vi "Modbus Slave Simple.vi"() -> ()   [LabVIEW 2017]
uses:
  <vilib>/NI/Modbus Library/API/Wrapper/Create Serial Slave.vi
  <vilib>/NI/Modbus Library/API/Slave/Modbus Slave.lvclass
  <vilib>/NI/Modbus Library/API/Wrapper/API Main.lvlib
panel:
  out "Array 5":errorcluster[](array[cluster])
  in  "Inputs":T1(array[cluster])=[{"Inputs"=[0, 0, 0, 0], "Address"=0, "Number"=4}] {"Inputs" scale=0.0..65535.0}
  out "error out":errorcluster
  in  "Stop Button":bool
  in  "Start":bool
  out "Array 4":errorcluster[](array[cluster])
  out "Array 3":errorcluster[](array[cluster])
  out "Array 2":errorcluster[](array[cluster])
  out "Array":errorcluster[](array[cluster])
  in  "Write Holding Reg":T2(array[cluster])=[{"Registers"=[], "Address"=0, "Number"=2}]
  in  "Read Holding Reg":T2(array[cluster])=[{"Registers"=[0, 0], "Address"=0, "Number"=2}]
  in  "Discrete Inputs":T3(array[cluster])=[{"Inputs"=[TRUE, FALSE, TRUE, FALSE], "Address"=0, "Number"=4}]
  in  "Coils":T4(array[cluster])=[{"Coils"=[TRUE, TRUE, TRUE, TRUE, TRUE, FALSE, FALSE, FALSE], "Address"=0, "Number"=8}] {"Address" format="%x"}
  in  "Update Period(ms)":u64=200
  in  "baud rate":u32=9600
  in  "VISA resource name":refnum<visa-resource-name>="COM14"
  in  "unit ID":u8=1
  in  "serial type":enum16{"RTU", "ASCII"}(ring)=enum."ASCII"
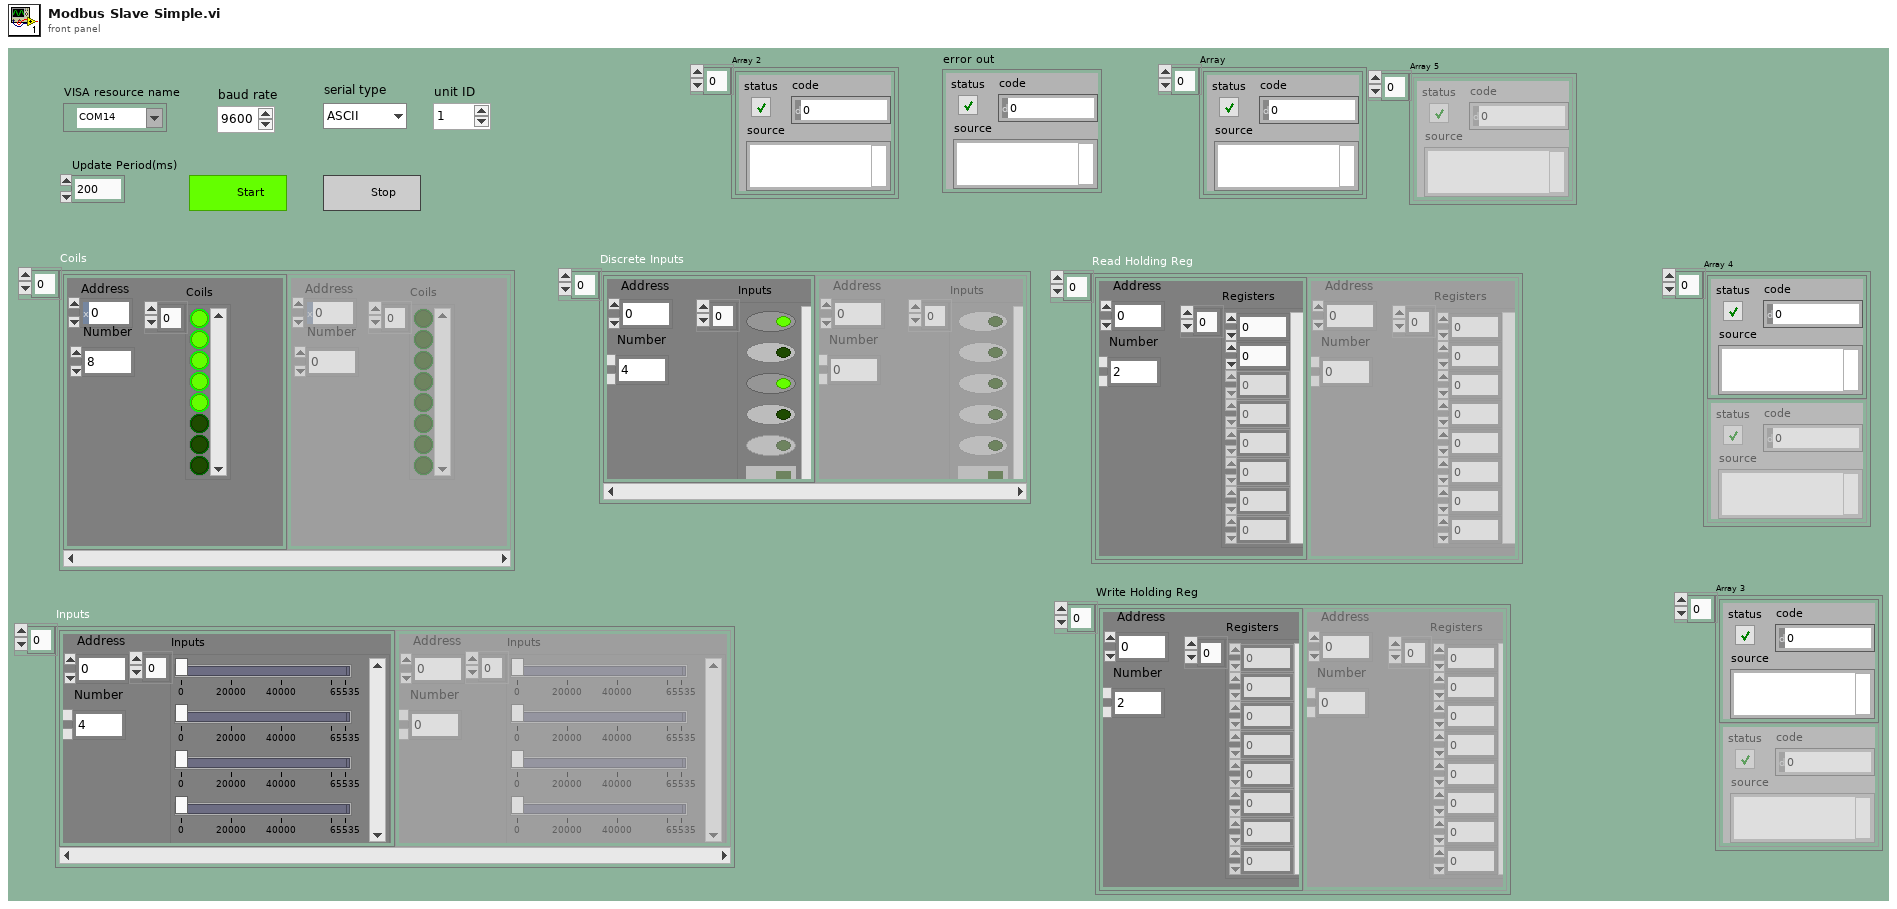
[diagram p1: front panel]
types:
  T1 = cluster{"Inputs":u16[], "Address":u16, "Number":u16}[]
  T2 = cluster{"Registers":u16[], "Address":u16, "Number":u16}[]
  T3 = cluster{"Inputs":bool[], "Address":u16, "Number":u16}[]
  T4 = cluster{"Coils":bool[], "Address":u16, "Number":u16}[]
  T5 = cluster{"Coils":bool[], "Address":u16, "Number":u16}
  T6 = cluster{"Registers":u16[], "Address":u16, "Number":u16}
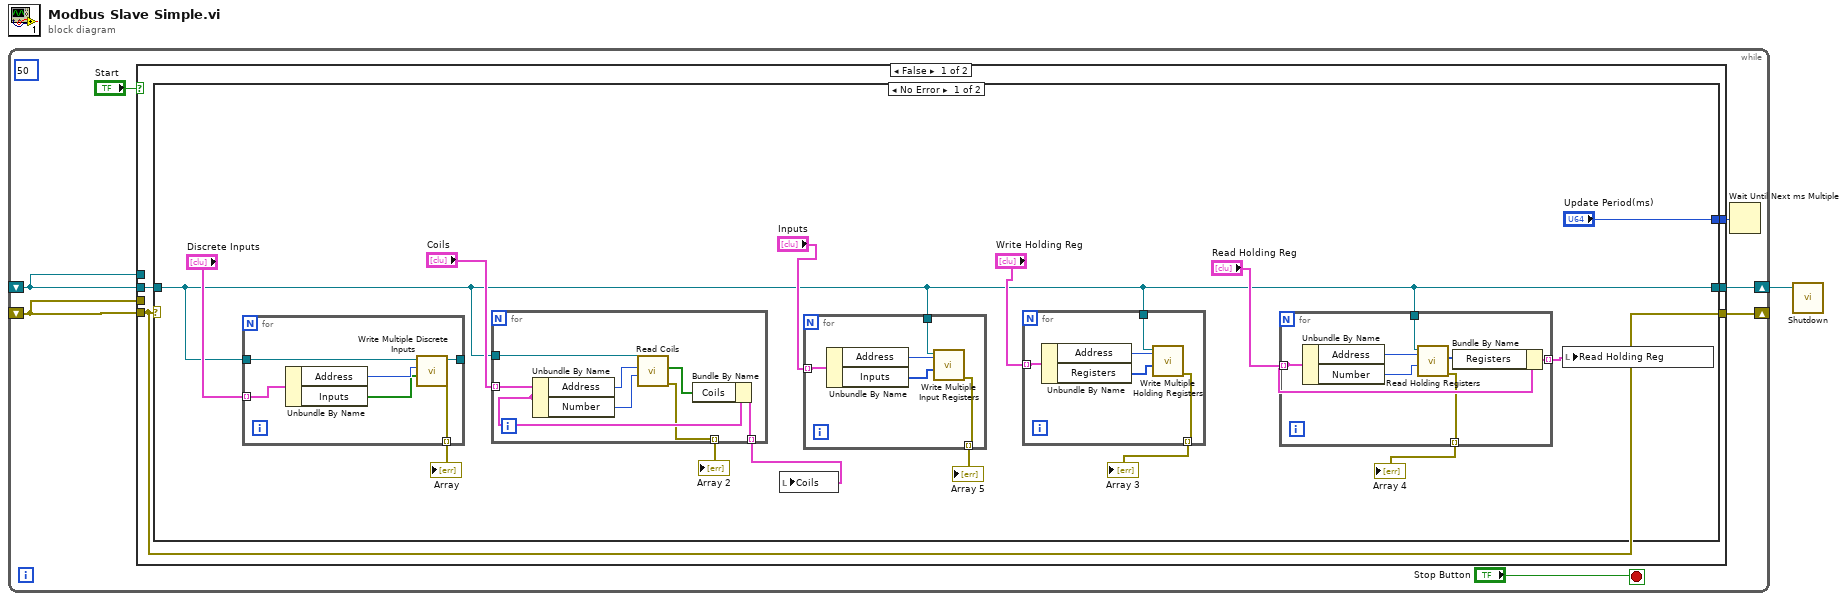
[diagram p0: block diagram]
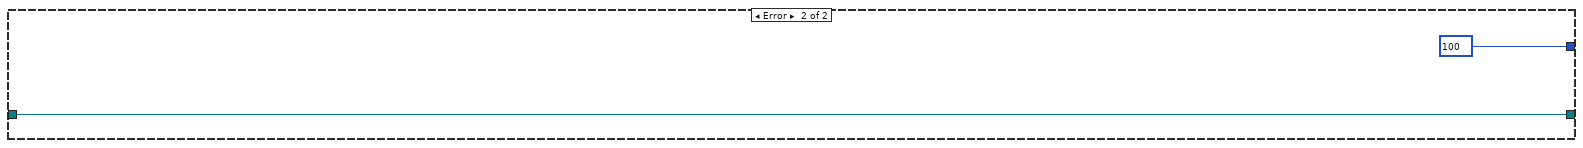
[diagram p2: hidden frame]
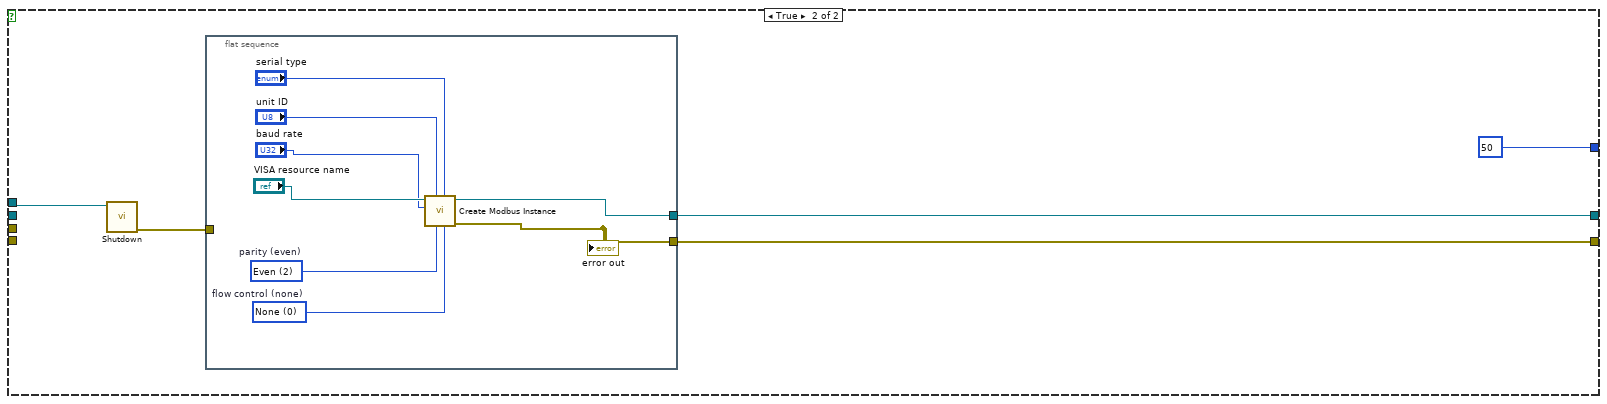
[diagram p3: hidden frame]
diagram:
  n1 = while {
    shift-right: [w6] -> w1
    shift-left: _ -> [w8]
    shift-right: [w5] -> _
    shift-left: _ -> [w7]
    stop <- "Stop Button" stop-if-true
    (unwired) 50
    n2 = case shown="False" "Start" {
      tunnel: w8 -> [w12 _]
      tunnel: w7 -> [w11 _]
      tunnel: w8 -> [_ w61]
      tunnel: w7 -> [_ _]
      tunnel: [w10 w63] -> w6
      tunnel: [w11 w62] -> w5
      tunnel: [w9 u64 50 ("Update Period(ms)")] -> w2
      frame False {
        n3 = case shown="No Error" w11 {
          tunnel: w12 -> [w14 w58]
          tunnel: [w14 w58] -> w10
          tunnel: ["Update Period(ms)" u64 100 ("Update Period(ms)")] -> w9
          frame No Error {
            n4 = for {
              tunnel: w14 -> [w56]
              tunnel: "Discrete Inputs" -> [w55] mode=indexing
              tunnel: [w52] -> _
              tunnel: [w51] -> w20 mode=indexing
              n5 = Unbundle By Name(w55) -> ("Address"=w54:u16, "Inputs"=w53:bool[])
              n6 = call-dynamic "Write Multiple Discrete Inputs.vi"("discrete inputs to write"=w53, "starting address"=w54, "Modbus slave in"=w56) -> ("error out"=w51:errorcluster, "Modbus slave out"=w52:refnum<class "Modbus Slave.lvclass">)  [unwired: 7 in]
            }
            "Array" <- w20
            n7 = for {
              tunnel: w14 -> [w50]
              tunnel: "Coils" -> [w48] mode=indexing
              tunnel: [w46] -> w16 mode=indexing
              tunnel: [w44] -> w19 mode=indexing
              n8 = Unbundle By Name(w48) -> ("Address"=w49:u16, "Number"=w45:u16)
              n9 = call-dynamic "Read Coils.vi"("number of inputs"=w45, "starting address"=w49, "Modbus slave in"=w50) -> ("error out"=w44:errorcluster, "coils"=w47:bool[])  [unwired: 6 in, 1 out]
              n10 = Bundle By Name(cluster=w48, "Coils"=w47) -> (w46:T5)
            }
            "Array 2" <- w19
            n11 = local write "Coils"(w16) -> ()
            n12 = for {
              tunnel: "Inputs" -> [w31] mode=indexing
              tunnel: [w28] -> w13 mode=indexing
              tunnel: w14 -> [w27]
              n13 = Unbundle By Name(w31) -> ("Address"=w30:u16, "Inputs"=w29:u16[])
              n14 = call-dynamic "Write Multiple Input Registers.vi"("input registers to write"=w29, "starting address"=w30, "Modbus slave in"=w27) -> ("error out"=w28:errorcluster)  [unwired: 7 in, 1 out]
            }
            "Array 5" <- w13
            n15 = for {
              tunnel: "Write Holding Reg" -> [w43] mode=indexing
              tunnel: w14 -> [w40]
              tunnel: [w39] -> w18 mode=indexing
              n16 = Unbundle By Name(w43) -> ("Address"=w42:u16, "Registers"=w41:u16[])
              n17 = call-dynamic "Write Multiple Holding Registers.vi"("registers to write"=w41, "starting address"=w42, "Modbus slave in"=w40) -> ("error out"=w39:errorcluster)  [unwired: 7 in, 1 out]
            }
            "Array 3" <- w18
            n18 = for {
              tunnel: "Read Holding Reg" -> [w35] mode=indexing
              tunnel: w14 -> [w37]
              tunnel: [w33] -> w23 mode=indexing
              tunnel: [w32] -> w17 mode=indexing
              n19 = Unbundle By Name(w35) -> ("Address"=w38:u16, "Number"=w36:u16)
              n20 = call-dynamic "Read Holding Registers.vi"("number of inputs"=w36, "starting address"=w38, "Modbus slave in"=w37) -> ("error out"=w32:errorcluster, "register values"=w34:u16[])  [unwired: 6 in, 1 out]
              n21 = Bundle By Name(cluster=w35, "Registers"=w34) -> (w33:T6)
            }
            "Array 4" <- w17
            n22 = local write "Read Holding Reg"(w23) -> ()
          }
          frame Error {
          }
        }
      }
      frame True {
        n23 = call-dynamic "Shutdown.vi"("Modbus slave in"=w61) -> ("error out"=w60:errorcluster)  [unwired: 10 in]
        n24 = flat-sequence {
          tunnel: [w71] -> w63
          tunnel: [w70] -> w62
          tunnel: w60 -> [_]
          frame #0 {
            w64 = u16 0 items=["None", "XON/XOFF", "RTS/CTS", "XON/XOFF & RTS/CTS", "DTR/DSR", "XON/XOFF & DTR/DSR"]  # flow control (none)
            w65 = u16 2 items=["None", "Odd", "Even", "Mark", "Space"]  # parity (even)
            n25 = call-poly <vilib>:"Create Modbus Instance.vi"("flow control"=w64, "serial type"="serial type", "parity (even)"=w65, "unit ID"="unit ID", "baud rate (9600)"="baud rate", "VISA resource name"="VISA resource name") -> ("error out"=w70:errorcluster, "serial slave instance"=w71:refnum<class "Modbus Slave.lvclass">)  [unwired: 4 in]
            "error out" <- w70
          }
        }
      }
    }
    n26 = Wait Until Next ms Multiple(millisecond multiple=w2) -> ()  [unwired: 1 out]
  }
  n27 = call-dynamic "Shutdown.vi"("Modbus slave in"=w1) -> ()  [unwired: 10 in, 1 out]
